vi "Set Output State.vi"(8 "error in (no error)":errorcluster, 10 "Output State":bool, 11 "Cooler in":refnum<class "Cooler.lvclass">) -> (0 "error out":errorcluster, 3 "Cooler out":refnum<class "Cooler.lvclass">)   [LabVIEW 2012, in "Cooler.lvlib" / "Cooler.lvclass"]
uses:
  Cooler.lvclass
  Cooler.lvclass/Cooler.ctl
  Cooler UI/Cooler UI with Events Messages/Update Pump Msg/Update Pump Msg.lvclass/Update Pump Msg.ctl
  <vilib>/ActorFramework/Message Enqueuer/Message Enqueuer.lvclass/Message Enqueuer.ctl
  <vilib>/ActorFramework/Time-Delayed Send Message/Time-Delay Override Options.ctl
  Dual Controller/Dual Fan Messages/Power On Msg/Power On Msg.lvclass
  <vilib>/ActorFramework/Message Enqueuer/Enqueue.vi
  Simulation/Simulation Data_Global.vi
  <vilib>/ActorFramework/Message Priority Queue/Priority Enqueue.vi
  Cooler UI/Cooler UI with Events Messages/Update Pump Msg/Update Pump Msg.lvclass
  Dual Controller/Dual Fan Messages/Power Off Msg/Power Off Msg.lvclass
  Simulation/Simulation.lvlib
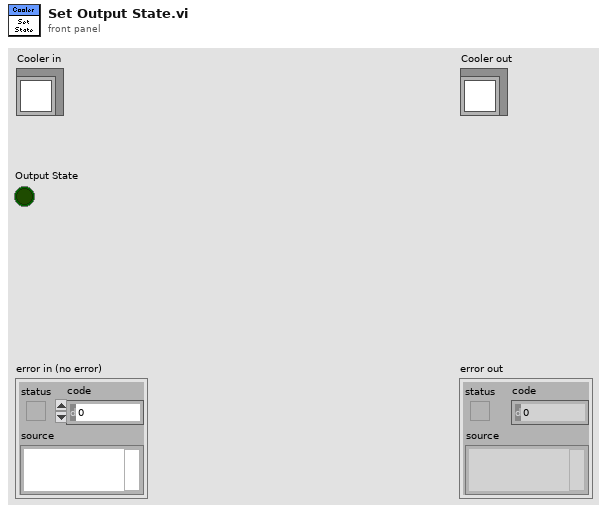
[diagram p1: front panel]
types:
  T1 = typedef "Time-Delay Override Options.ctl" = enum16{"Send next copy now", "Skip next scheduled copy", "Send next copy now and stop all further copies", "Stop all further copies"}
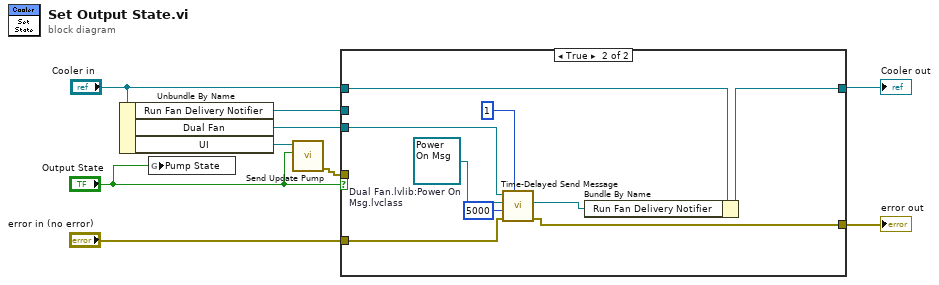
[diagram p0: block diagram]
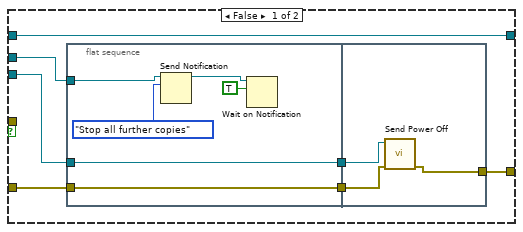
[diagram p2: hidden frame]
diagram:
  n1 = Unbundle By Name("Cooler in") -> ("Run Fan Delivery Notifier"=w7:refnum<notifier>, "Dual Fan"=w5:refnum<class "Message Enqueuer.lvclass">, "UI"=w3:refnum<class "Message Enqueuer.lvclass">)
  n2 = global write "Simulation Data_Global.vi" "Pump State"("Output State") -> ()
  n3 = call "Send Update Pump.vi"("Pump State"="Output State", "Message Enqueuer"=w3) -> ("error out"=w1:errorcluster)  [unwired: 8 in, 1 out]
  n4 = case shown="True" "Output State" {
    tunnel: "error in (no error)" -> [w14 w26]
    tunnel: "Cooler in" -> [w16 w34]
    tunnel: [w16 w33] -> w8
    tunnel: w7 -> [w13 _]
    tunnel: w5 -> [w12 w32]
    tunnel: [w10 w27] -> w4
    tunnel: w1 -> [_ _]
    frame False {
      n5 = flat-sequence {
        tunnel: w13 -> [w21]
        tunnel: [w22] -> w15
        tunnel: w14 -> [w22]
        tunnel: w12 -> [w17]
        tunnel: [w17] -> w11
        tunnel: w15 -> [w24]
        tunnel: w11 -> [w25]
        tunnel: [w23] -> w10
        frame #0 {
          n6 = Send Notification(notification=Time-Delay_Override_Options."Stop all further copies", notifier=w21) -> (notifier out=w19:refnum<notifier>)  [unwired: 1 in, 1 out]
          n7 = Wait on Notification(notifier=w19, ignore previous (F)=TRUE) -> ()  [unwired: 2 in, 4 out]
        }
        frame #1 {
          n8 = call "Send Power Off.vi"("error in (no error)"=w24, "Message Enqueuer"=w25) -> ("error out"=w23:errorcluster)  [unwired: 8 in, 1 out]
        }
      }
    }
    frame True {
      w30 = refnum<class "Power On Msg.lvclass"> refnum  # Dual Fan.lvlib:Power On Msg.lvclass
      n9 = call <vilib>:"Time-Delayed Send Message.vi"("# Copies (0 = infinite repeat)"=u32 1, "error in (no error)"=w26, "Milliseconds To Wait"=5000, "Message"=w30, "Message Enqueuer"=w32) -> ("error out"=w27:errorcluster, "Delivery Notifier"=w28:refnum<notifier>)  [unwired: 5 in]
      n10 = Bundle By Name(cluster=w34, "Run Fan Delivery Notifier"=w28) -> (w33:refnum<class "Cooler.lvclass">)
    }
  }
  "error out" <- w4
  "Cooler out" <- w8
